vi "Event handler-Funct Acq button.vi"(11 "Funct.Acq button's value":bool) -> (0 "error out":errorcluster)   [LabVIEW 2020]
uses:
  Typedefs/Set Main VI cursor.ctl
  Typedefs/Top level VI states.ctl
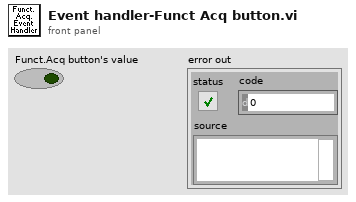
[diagram p1: front panel]
types:
  T1 = typedef "Set Main VI cursor.ctl" = enum16{"Release busy cursor", "Set busy cursor"}
  T2 = typedef "Top level VI states.ctl" = enum16{"None", "Initialise UI", "<STACK PROTOCOL STATES>", "AOL Zstack-START", "AOL Zstack-STOP", "Motor Zstack-START", "Motor Zstack-STOP", "<ACQUISITION PROTOCOL STATES> ", "Functional Acquisition-START", "Functional Acquisition-STOP", "Single Plane Acquisition-START", "Single Plane Acquisition-STOP", "Volume Acquisition-START", "Volume Acquisition-STOP", "<LIVE IMAGING PROTOCOL STATES>", "Live Imaging-START", "Live Imaging-STOP", "Live Plane Imaging-START", "Live Plane Imaging-STOP", "Live Volume Imaging-START", "Live Volume Imaging-STOP", "<MOVEMENT CORRECTION PROTOCOL STATES>", "EXIT"}
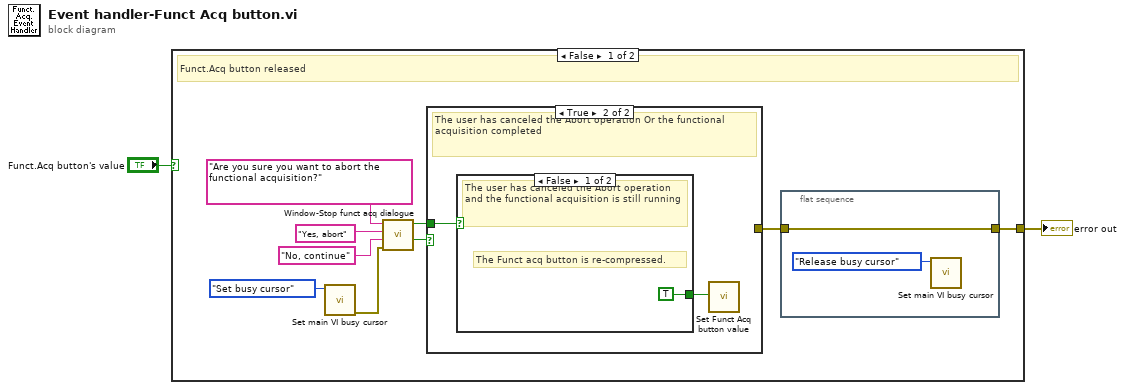
[diagram p0: block diagram]
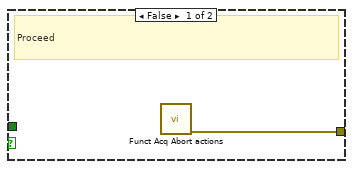
[diagram p2: hidden frame]
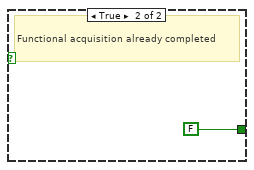
[diagram p3: hidden frame]
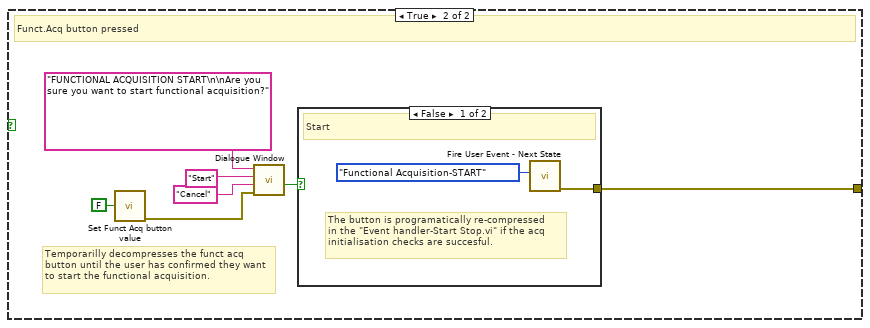
[diagram p4: hidden frame]
diagram:
  n1 = case shown="False" "Funct.Acq button's value" {
    tunnel: [w3 w25] -> w1
    frame False {
      # "Funct.Acq button released"
      n2 = call "Set main VI busy cursor.vi"("Main VI's cursor"=Set_Main_VI_cursor."Set busy cursor") -> ("error out"=w5:errorcluster)  [unwired: 10 in]
      n3 = call "Window-Stop funct acq dialogue.vi"("error in (no error)"=w5, "Caption-Left button (Cancel)"="No, continue", "Caption-Right button (OK)"="Yes, abort", "Message string"="Are you sure you want to abort the functional acquisition?") -> ("User canceled the Abort Or the func acqcompleted"=w11:bool, "Funct acq completed"=w7:bool)  [unwired: 5 in, 1 out]
      n4 = case shown="True" w11 {
        tunnel: [w14 _] -> w4
        tunnel: w7 -> [_ w16]
        frame False {
          # "Proceed"
          n5 = call "Funct Acq Abort actions.vi"() -> ("error out"=w14:errorcluster)  [unwired: 11 in]
        }
        frame True {
          # "The user has canceled the Abort operation Or the functional acquisition completed"
          n6 = case shown="False" w16 {
            tunnel: [TRUE ("Value") FALSE ("Value")] -> w15
            frame False {
              # "The Funct acq button is re-compressed."
              # "The user has canceled the Abort operation and the functional acquisition is still running"
            }
            frame True {
              # "Functional acquisition already completed"
            }
          }
          n7 = call "Set Funct Acq button value.vi"("Functional Acquisition button's new value"=w15) -> ()  [unwired: 10 in, 1 out]
        }
      }
      n8 = flat-sequence {
        tunnel: w4 -> [w12]
        tunnel: [w12] -> w3
        frame #0 {
          n9 = call "Set main VI busy cursor.vi"("Main VI's cursor"=Set_Main_VI_cursor."Release busy cursor") -> ()  [unwired: 10 in, 1 out]
        }
      }
    }
    frame True {
      # "Temporarilly decompresses the funct acq button until the user has confirmed they want to start the functional acquisition."
      # "Funct.Acq button pressed"
      n10 = call "Set Funct Acq button value.vi"("Functional Acquisition button's new value"=FALSE ("Value")) -> ("error out"=w19:errorcluster)  [unwired: 10 in]
      n11 = call "Dialogue Window.vi"("error in (no error)"=w19, "Caption-Left button (Cancel)"="Cancel", "Caption-Right button (OK)"="Start", "Message string"="FUNCTIONAL ACQUISITION START\n\nAre you sure you want to start functional acquisition?") -> ("Cancelled (Left button pressed)"=w21:bool)  [unwired: 5 in, 2 out]
      n12 = case shown="False" w21 {
        tunnel: [w26 _] -> w25
        frame False {
          # "The button is programatically re-compressed\nin the \"Event handler-Start Stop.vi\" if the acq\ninitialisation checks are succesful."
          # "Start"
          n13 = call "Fire User Event - Next State.vi"("\"UI Handler loop\" case to execute"=Top_level_VI_states."Functional Acquisition-START" ("event data / imaging mode")) -> ("Error Out"=w26:errorcluster)  [unwired: 10 in]
        }
        frame True {
          # "Cancelled"
        }
      }
    }
  }
  "error out" <- w1
